vi "Wire Error Case Structure for RCF.vi"(8 "error in (no error)":errorcluster, 11 "Vi Ref":refnum<vi>) -> (0 "error out":errorcluster)   [LabVIEW 2018]
uses:
  Scripting Tools.lvlib
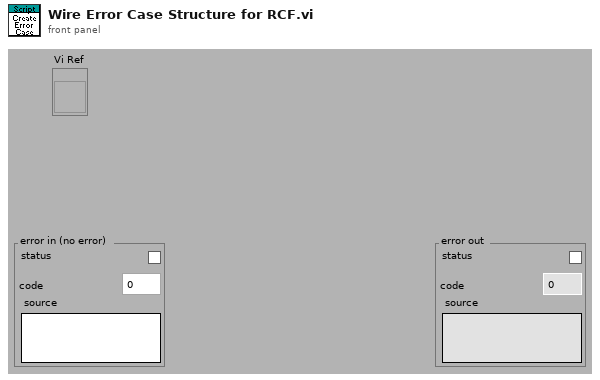
[diagram p1: front panel]
types:
  T1 = enum16{"Case Structure", "Stacked Sequence", "Event Structure", "Diagram Disable", "Conditional Disable", "While Loop", "For Loop"}
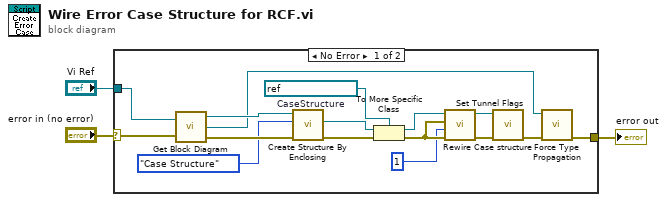
[diagram p0: block diagram]
diagram:
  n1 = case shown="No Error" "error in (no error)" {
    selector: "error in (no error)" -> [w7 w20]
    tunnel: [w8 w20] -> w3
    tunnel: "Vi Ref" -> [w6 _]
    frame No Error {
      w14 = refnum<vi> refnum  # CaseStructure
      n2 = call "Get Block Diagram.vi"("vi refnum in"=w6, "error in (no error)"=w7) -> ("Diagram"=w18:refnum<vi>, "vi refnum out"=w10:refnum<vi>, "error out"=w19:errorcluster)
      n3 = call "Create Structure By Enclosing.vi"("error in (no error)"=w19, "Structure Type"=T1."Case Structure", "Diagram In"=w18) -> ("error out"=w16:errorcluster, "Structure Out"=w15:refnum<vi>)  [unwired: 1 in, 6 out]
      n4 = To More Specific Class(target class=w14, reference=w15, error in=w16) -> (specific class reference=w13:refnum<vi>, error out=w5:errorcluster)
      n5 = call "Rewire Case structure.vi"("error in (no error)"=w5, "Wire All Cases Except this One ?"=1, "Selector Type"=w5, "CaseSel Refnum"=w13) -> ("error out"=w12:errorcluster, "CaseSel Refnum Out"=w11:refnum<vi>)  [unwired: 6 out]
      n6 = call "Set Tunnel Flags.vi"("error in (no error)"=w12, "Struct Refnum"=w11) -> ("error out"=w9:errorcluster)  [unwired: 9 out]
      n7 = call "Force Type Propagation.vi"("error in (no error)"=w9, "reference"=w10) -> ("error out"=w8:errorcluster)  [unwired: 1 in, 8 out]
    }
    frame Error {
    }
  }
  "error out" <- w3
